vi "List Roots.vi"(10 "Optional Root Name":string, 11 "Tree Map In":T1) -> (3 "Unique Root Paths Set":set{string}(c389))   [LabVIEW 2021, in "Tree Map.lvlib"]
doc: "Iterates through all tree nodes and finds the root nodes. This feature is designed only for the Tree Map, since an XML document cannot contain more than 1 root.\n\n<b>Author:</b> Piotr Kruczkowski <PrimaryKey>\n<b>License:</b> NewBSD\n\nCopyright (c) 2019, National Instruments\nAll rights reserved.\n\nRedistribution and use in source and binary forms, with or without\nmodification, are permitted provided that the following conditions are met:\n1. Redistributions of source code must retain the above copyright\n notice, this list of conditions and the following disclaimer.\n2. Redistributions in binary form must reproduce the above copyright\n notice, this list of conditions and the following disclaimer in the\n documentation and/or other materials provided with the distribution.\n3. Neither the name of National Instruments nor the\n names of its contributors may be used to endorse or promote products\n derived from this software without specific prior written permission.\n\nTHIS SOFTWARE IS PROVIDED BY National Instruments ''AS IS'' AND ANY\nEXPRESS OR IMPLIED WARRANTIES, INCLUDING, BUT NOT LIMITED TO, THE IMPLIED\nWARRANTIES OF MERCHANTABILITY AND FITNESS FOR A PARTICULAR PURPOSE ARE\nDISCLAIMED. IN NO EVENT SHALL National Instruments BE LIABLE FOR ANY\nDIRECT, INDIRECT, INCIDENTAL, SPECIAL, EXEMPLARY, OR CONSEQUENTIAL DAMAGES\n(INCLUDING, BUT NOT LIMITED TO, PROCUREMENT OF SUBSTITUTE GOODS OR SERVICES;\nLOSS OF USE, DATA, OR PROFITS; OR BUSINESS INTERRUPTION) HOWEVER CAUSED AND\nON ANY THEORY OF LIABILITY, WHETHER IN CONTRACT, STRICT LIABILITY, OR TORT\n(INCLUDING NEGLIGENCE OR OTHERWISE) ARISING IN ANY WAY OUT OF THE USE OF THIS\nSOFTWARE, EVEN IF ADVISED OF THE POSSIBILITY OF SUCH DAMAGE."
uses:
  <vilib>/National Instruments/Tree Map/Tree Map.lvlib
  <vilib>/National Instruments/Tree Map/Tree Map Data.ctl
  <vilib>/National Instruments/Tree Map/Utility/Join Strings Tree.vi
  <vilib>/National Instruments/Tree Map/SubVIs/TM Head and Tail.vi
  <vilib>/National Instruments/Tree Map/SubVIs/TM Init and Last.vi
  <vilib>/National Instruments/Tree Map/Utility/Split String Tree.vi
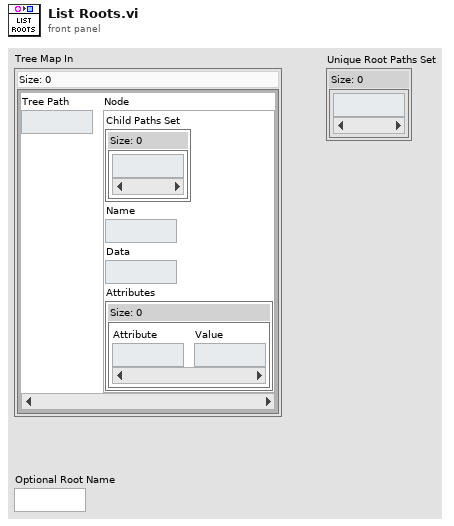
[diagram p1: front panel]
types:
  T1 = typedef "Tree Map.lvlib/Tree Map Data.ctl" = map{string, cluster{"Child Paths Set":set{string}, "Name":string, "Data":string, "Attributes":map{string, string}}}
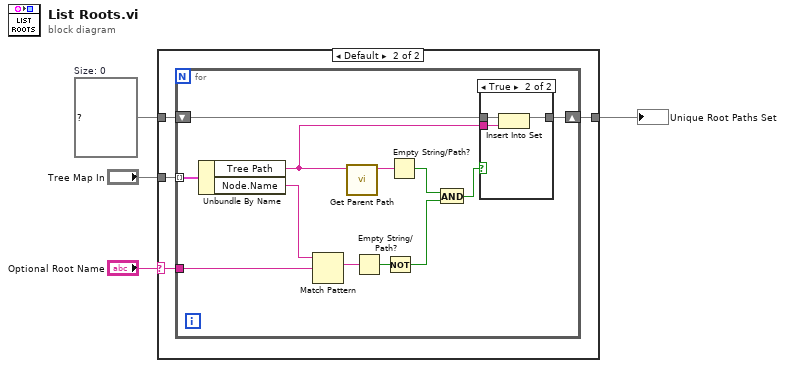
[diagram p0: block diagram]
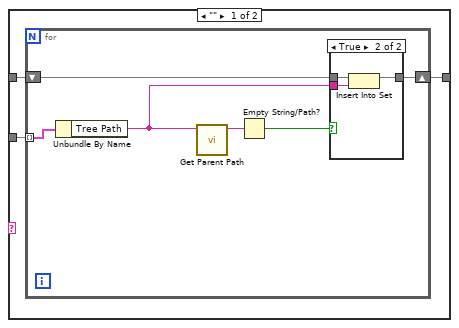
[diagram p2: hidden frame]
diagram:
  w3 = set{string} {}  # Size: 0
  n1 = case shown="Default" "Optional Root Name" {
    selector: "Optional Root Name" -> [_ w18]
    tunnel: "Tree Map In" -> [w5 w21]
    tunnel: w3 -> [w7 w20]
    tunnel: [w6 w19] -> w2
    frame "" {
      n2 = for {
        tunnel: w5 -> [w13] mode=indexing
        shift-right: [w10] -> w6
        shift-left: w7 -> [w9]
        n3 = Unbundle By Name(w13) -> ("Tree Path"=w11:string)
        n4 = call <vilib>:"Get Parent Path.vi"("Node Path"=w11) -> ("Parent Path"=w12:string)  [unwired: 8 in, 2 out]
        n5 = Empty String/Path?(string/path=w12) -> (empty?=w8:bool)
        n6 = case shown="True" w8 {
          tunnel: w11 -> [_ w17]
          tunnel: [w14 w16] -> w10
          tunnel: w9 -> [w14 w15]
          frame False {
          }
          frame True {
            n7 = Insert Into Set(10:w17, 11:w15) -> (3:w16:set{string})  [unwired: 1 out]
          }
        }
      }
    }
    frame Default {
      n8 = for {
        tunnel: w21 -> [w33] mode=indexing
        shift-right: [w30] -> w19
        shift-left: w20 -> [w29]
        tunnel: w18 -> [w27]
        n9 = Unbundle By Name(w33) -> ("Tree Path"=w31:string, "Node.Name"=w26:string)
        n10 = Match Pattern(string=w26, regular expression=w27) -> (match substring=w28:string)  [unwired: 1 in, 3 out]
        n11 = call <vilib>:"Get Parent Path.vi"("Node Path"=w31) -> ("Parent Path"=w32:string)  [unwired: 8 in, 2 out]
        n12 = Empty String/Path?(string/path=w28) -> (empty?=w24:bool)
        n13 = Not(x=w24) -> (.not. x?=w22:bool)
        n14 = Empty String/Path?(string/path=w32) -> (empty?=w25:bool)
        n15 = And(x=w25, y=w22) -> (x .and. y?=w23:bool)
        n16 = case shown="True" w23 {
          tunnel: w31 -> [_ w37]
          tunnel: [w34 w36] -> w30
          tunnel: w29 -> [w34 w35]
          frame False {
          }
          frame True {
            n17 = Insert Into Set(10:w37, 11:w35) -> (3:w36:set{string})  [unwired: 1 out]
          }
        }
      }
    }
  }
  "Unique Root Paths Set" <- w2
